vi "execution class name.vi"(8 "error in":errorcluster, 11 "My Awesome Control Modules configuration in":refnum<class "My Awesome Control Modules configuration.lvclass">) -> (0 "error out":errorcluster, 2 "class name":string, 3 "My Awesome Control Modules configuration out":refnum<class "My Awesome Control Modules configuration.lvclass">)   [LabVIEW 2013, in "My Awesome Control Modules configuration.lvclass"]
doc: "Provides an interface for determining the module runtime class associated with this module configuration. This class name can then be used to dynamically load or locate the runtime class for initialization purposes."
uses:
  My Awesome Control Modules configuration.lvclass
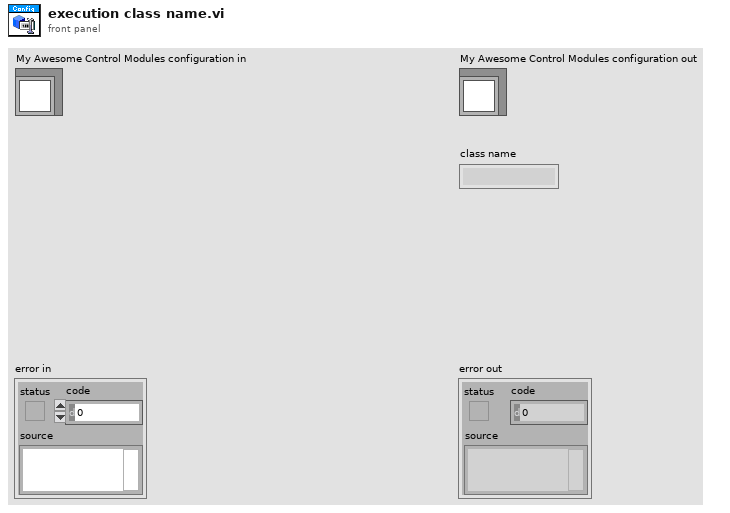
[diagram p1: front panel]
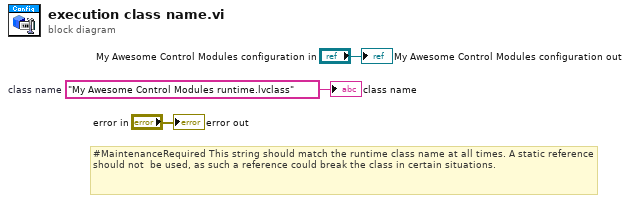
[diagram p0: block diagram]
diagram:
  w1 = "My Awesome Control Modules runtime.lvclass"  # class name
  # "#MaintenanceRequired This string should match the runtime class name at all times. A static reference should not  be used, as such a reference could break the class in certain situations."
  "error out" <- "error in"
  "My Awesome Control Modules configuration out" <- "My Awesome Control Modules configuration in"
  "class name" <- w1
